vi "NTCP Propose 2 Targets.vi"(2 "error in":errorcluster, 3 "Payload":T1[](array[typedef])) -> (0 "error out":errorcluster, 1 "Step Out":T3[](array[typedef]))   [LabVIEW 2009]
uses:
  MixedMode/Widget/Target.ctl
  Data Access Objects/Metadata/LBCB Number.ctl
  NTCP library/Payload.ctl
  Control Point Suffix.ctl
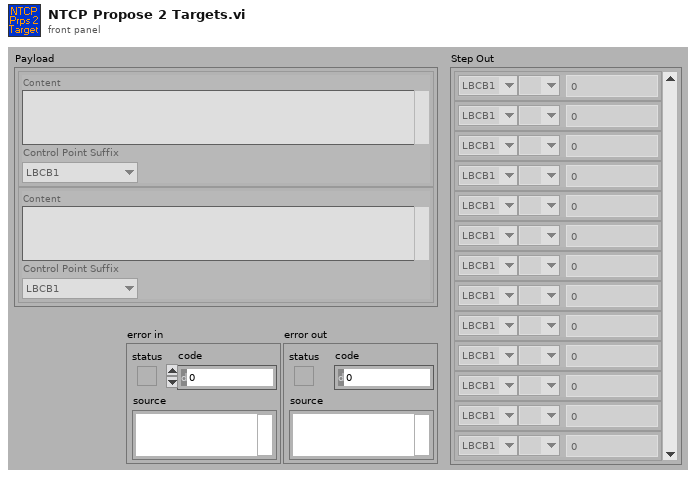
[diagram p1: front panel]
types:
  T1 = typedef "Payload.ctl" = cluster{"Content":string, "Control Point Suffix":T2}
  T2 = typedef "Control Point Suffix.ctl" = enum16{"LBCB1", "LBCB2", "ExternalSensors"}
  T3 = typedef "Target.ctl" = cluster{"LBCB Number":T4, "DOF Vectors":enum16{" ", "Dx", "Dy", "Dz", "Rx", "Ry", "Rz", "Fx", "Fy", "Fz", "Mx", "My", "Mz"}, "Amount":dbl}
  T4 = typedef "LBCB Number.ctl" = enum16{"LBCB1", "LBCB2"}
  T5 = typedef "Propose Command.ctl" = cluster{"Control Type":i32[], "Value":dbl[]}
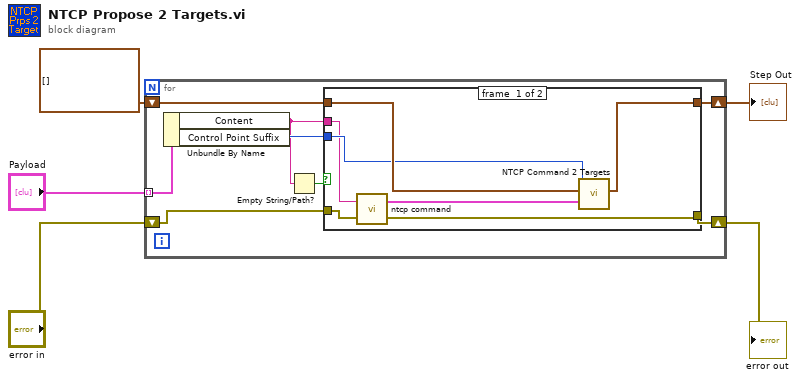
[diagram p0: block diagram]
diagram:
  n1 = for {
    shift-right: [w12] -> w3
    shift-left: T3[] [] ("Step Out") -> [w13]
    tunnel: "Payload" -> [w11] mode=indexing
    shift-right: [w6] -> w5
    shift-left: "error in" -> [w7]
    n2 = Unbundle By Name(w11) -> ("Content"=w8:string, "Control Point Suffix"=w10:T2)
    n3 = Empty String/Path?(string/path=w8) -> (empty?=w9:bool)
    n4 = case shown="False" w9 {
      tunnel: w13 -> [w19 w22]
      tunnel: [w16 w22] -> w12
      tunnel: w10 -> [w18 _]
      tunnel: w8 -> [w17 _]
      tunnel: w7 -> [w15 w21]
      tunnel: [w14 w21] -> w6
      frame #0 {
        n5 = call "ntcp command.vi"("error in"=w15, "Input string"=w17) -> ("Error out"=w14:errorcluster, "NTCP Command"=w20:T5)
        n6 = call "NTCP Command 2 Targets.vi"("NTCP Command"=w20, "Targets In"=w19, "Contol\nPoint\nSuffix"=w18) -> ("Targets Out"=w16:T3[])  [unwired: 8 out]
      }
      frame #1 {
      }
    }
  }
  "error out" <- w5
  "Step Out" <- w3
